vi "Configuration.vi"() -> ()   [LabVIEW 2018]
uses:
  <vilib>/Utility/miscctls.llb/LVRectTypeDef.ctl
  <vilib>/addons/database/NI_Database_API.lvlib
panel:
  in  "View":bool
  out "Headline":string
  in  "Delete Button":bool
  in  "Save Button":bool
  in  "Configuration":T1
  in  "Remark":string
  in  "Project ID":string(combo) caption="Test Name"
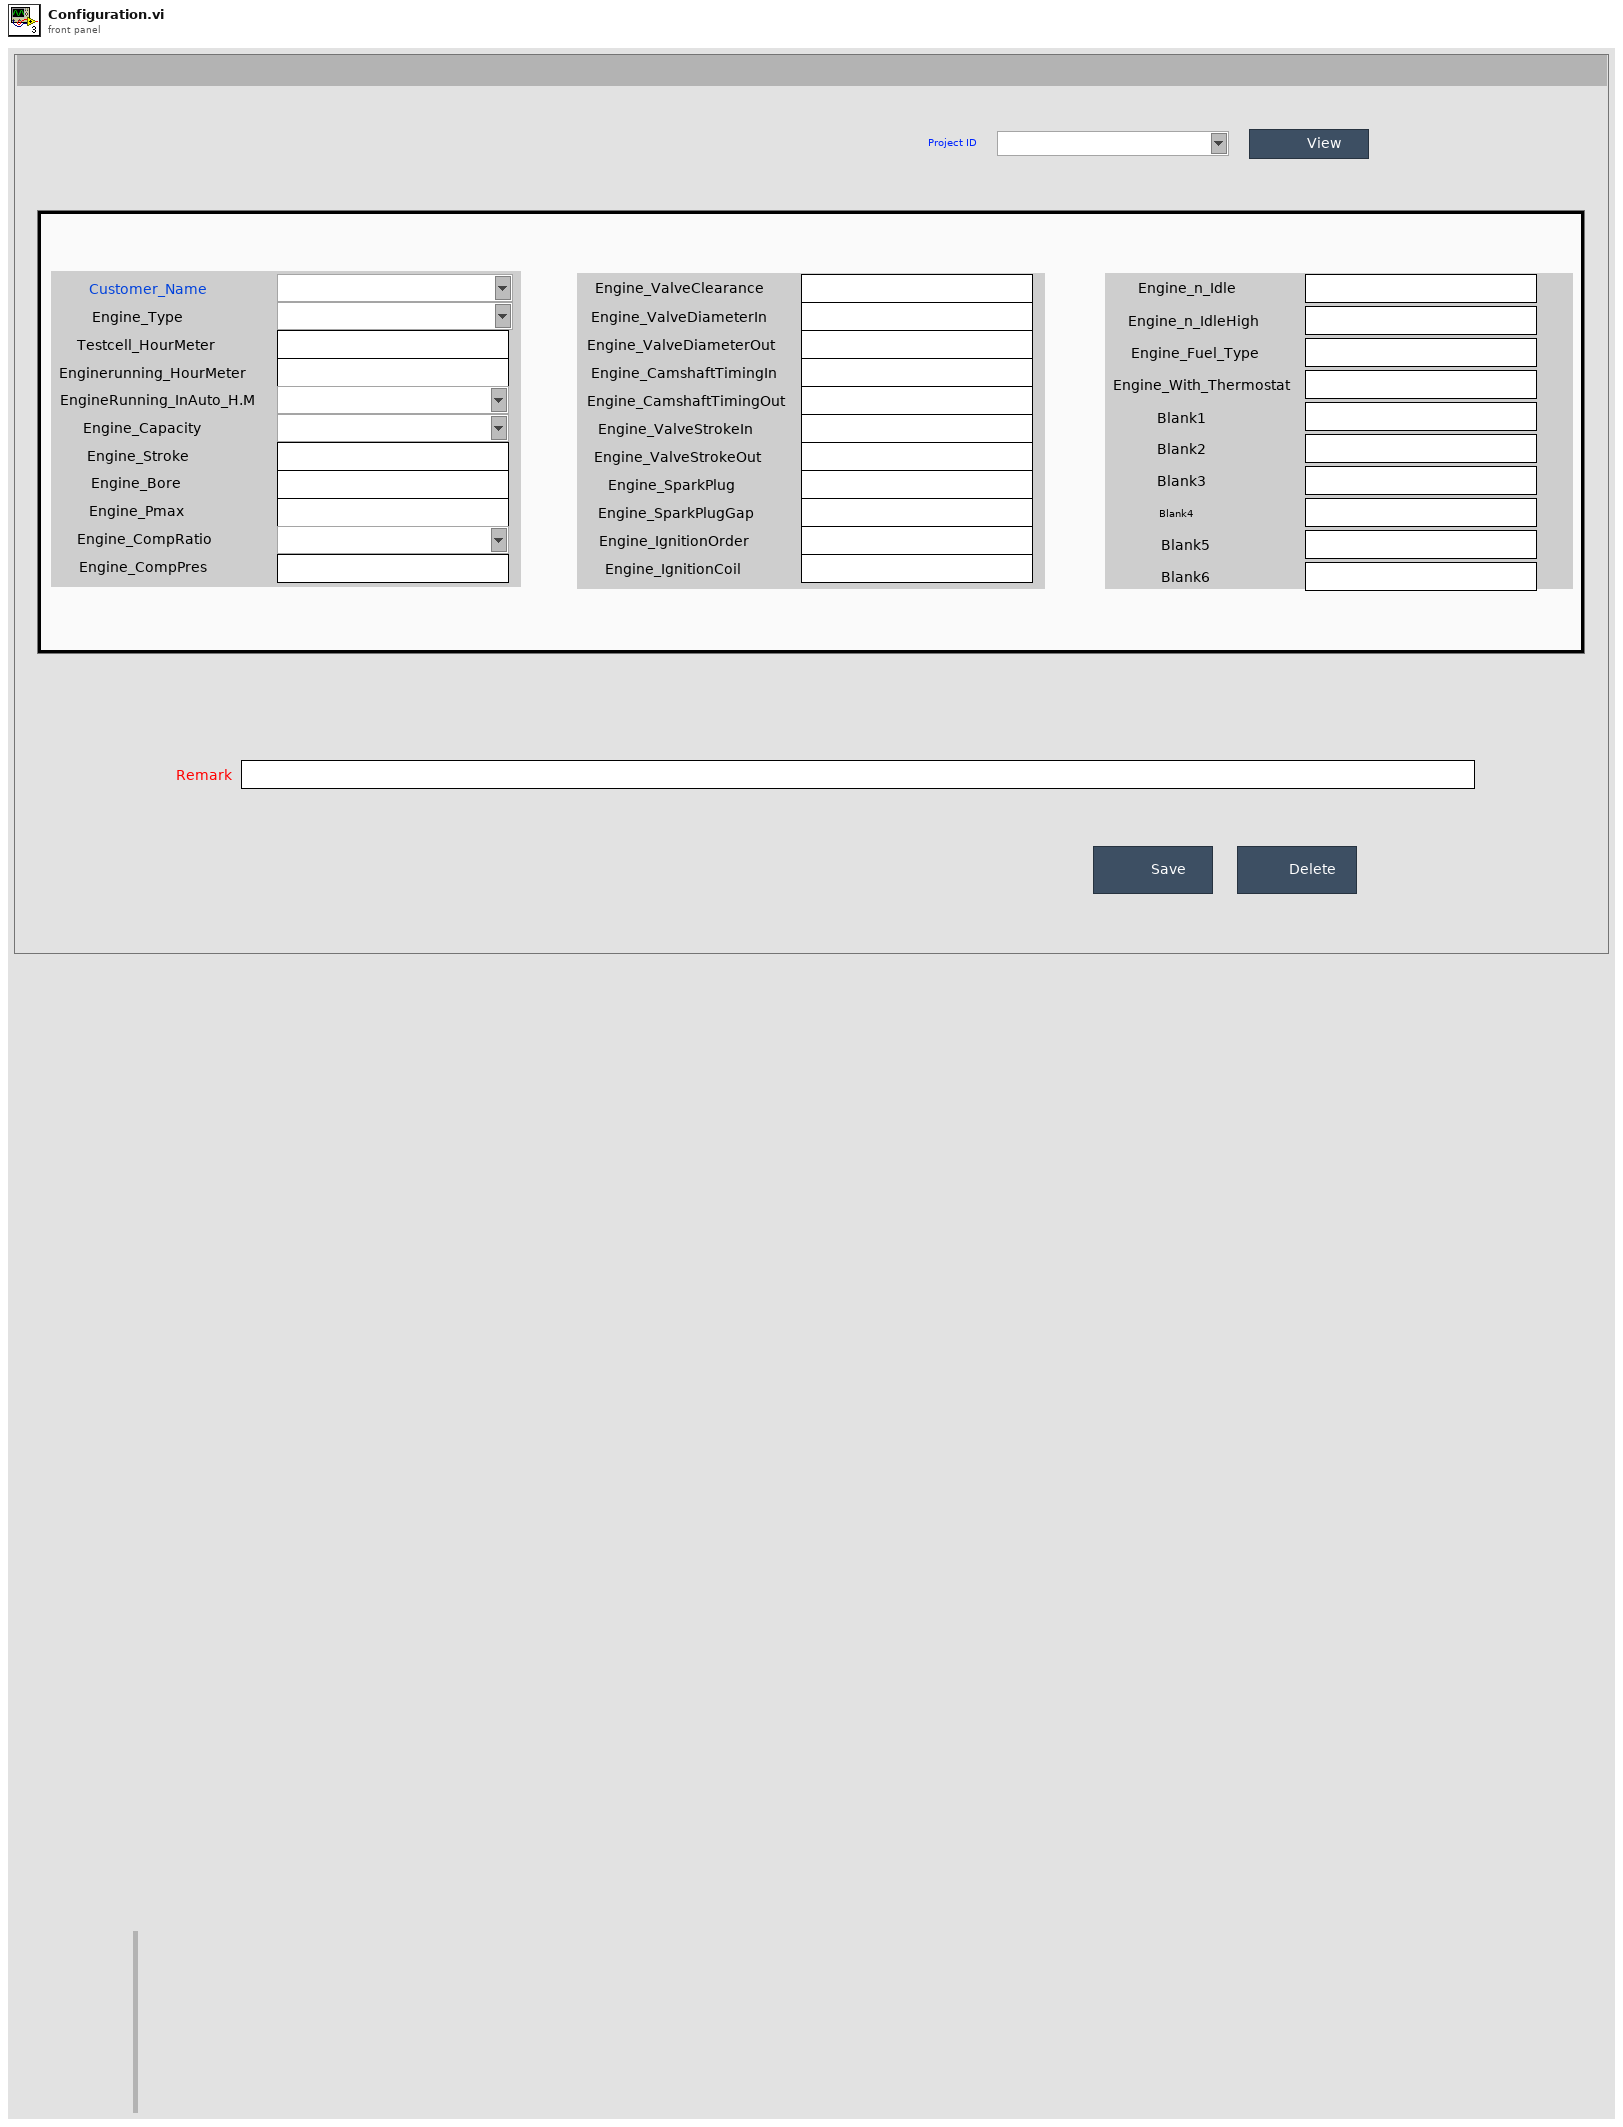
[diagram p1: front panel]
types:
  T1 = cluster{"Customer_Name":string, "Engine_Type":string, "Testcell_HourMeter":string, "Enginerunning_HourMeter":string, "EngineRunning_InAuto_H.M":string, "Engine_Capacity":string, "Engine_Stroke":string, "Engine_Bore":string, "Engine_Pmax":string, "Engine_CompRatio":string, "Engine_CompPres":string, "Engine_ValveClearance":string, "Engine_ValveDiameterIn":string, "Engine_ValveDiameterOut":string, "Engine_CamshaftTimingIn":string, "Engine_CamshaftTimingOut":string, "Engine_ValveStrokeIn":string, "Engine_ValveStrokeOut":string, "Engine_SparkPlug":string, "Engine_SparkPlugGap":string, "Engine_IgnitionOrder":string, "Engine_IgnitionCoil":string, "Engine_n_Idle":string, "Engine_n_IdleHigh":string, "Engine_Fuel_Type":string, "Engine_With_Thermostat":string, "Blank1":string, "Blank2":string, "Blank3":string, "Blank4":string, "Blank5":string, "Blank6":string}
  T2 = enum32{"Invalid", "Standard", "Closed", "Hidden", "Minimized", "Maximized"}
  T3 = enum32{"invalid app kind", "Development System", "Run Time System", "Student Edition", "Embedded LabVIEW", "Evaluation", "Custom"}
  T4 = typedef "LVRectTypeDef.ctl" = cluster{"Left":i16, "Top":i16, "Right":i16, "Bottom":i16}
  T5 = typedef "NI_Database_API.lvlib/Conn ObjectReference.ctl" = refnum<k1>
  T6 = cluster{"Core":cluster{"Current VI Reference":refnum<vi>, "Close Panel on Exit?":bool}, "Project ID":refnum<vi>, "Remark":refnum<vi>, "Controls[]":refnum<vi>[], "connection reference":T5}
  T7 = cluster{"Current VI Reference":refnum<vi>, "Close Panel on Exit?":bool}
  T8 = cluster{"[0]":string, "[1]":string, "[2]":string, "[3]":string, "[4]":string, "[5]":string, "[6]":string, "[7]":string, "[8]":string, "[9]":string, "[10]":string, "[11]":string, "[12]":string, "[13]":string, "[14]":string, "[15]":string, "[16]":string, "[17]":string, "[18]":string, "[19]":string, "[20]":string, "[21]":string, "[22]":string, "[23]":string, "[24]":string, "[25]":string, "[26]":string, "[27]":string, "[28]":string, "[29]":string, "[30]":string, "[31]":string}
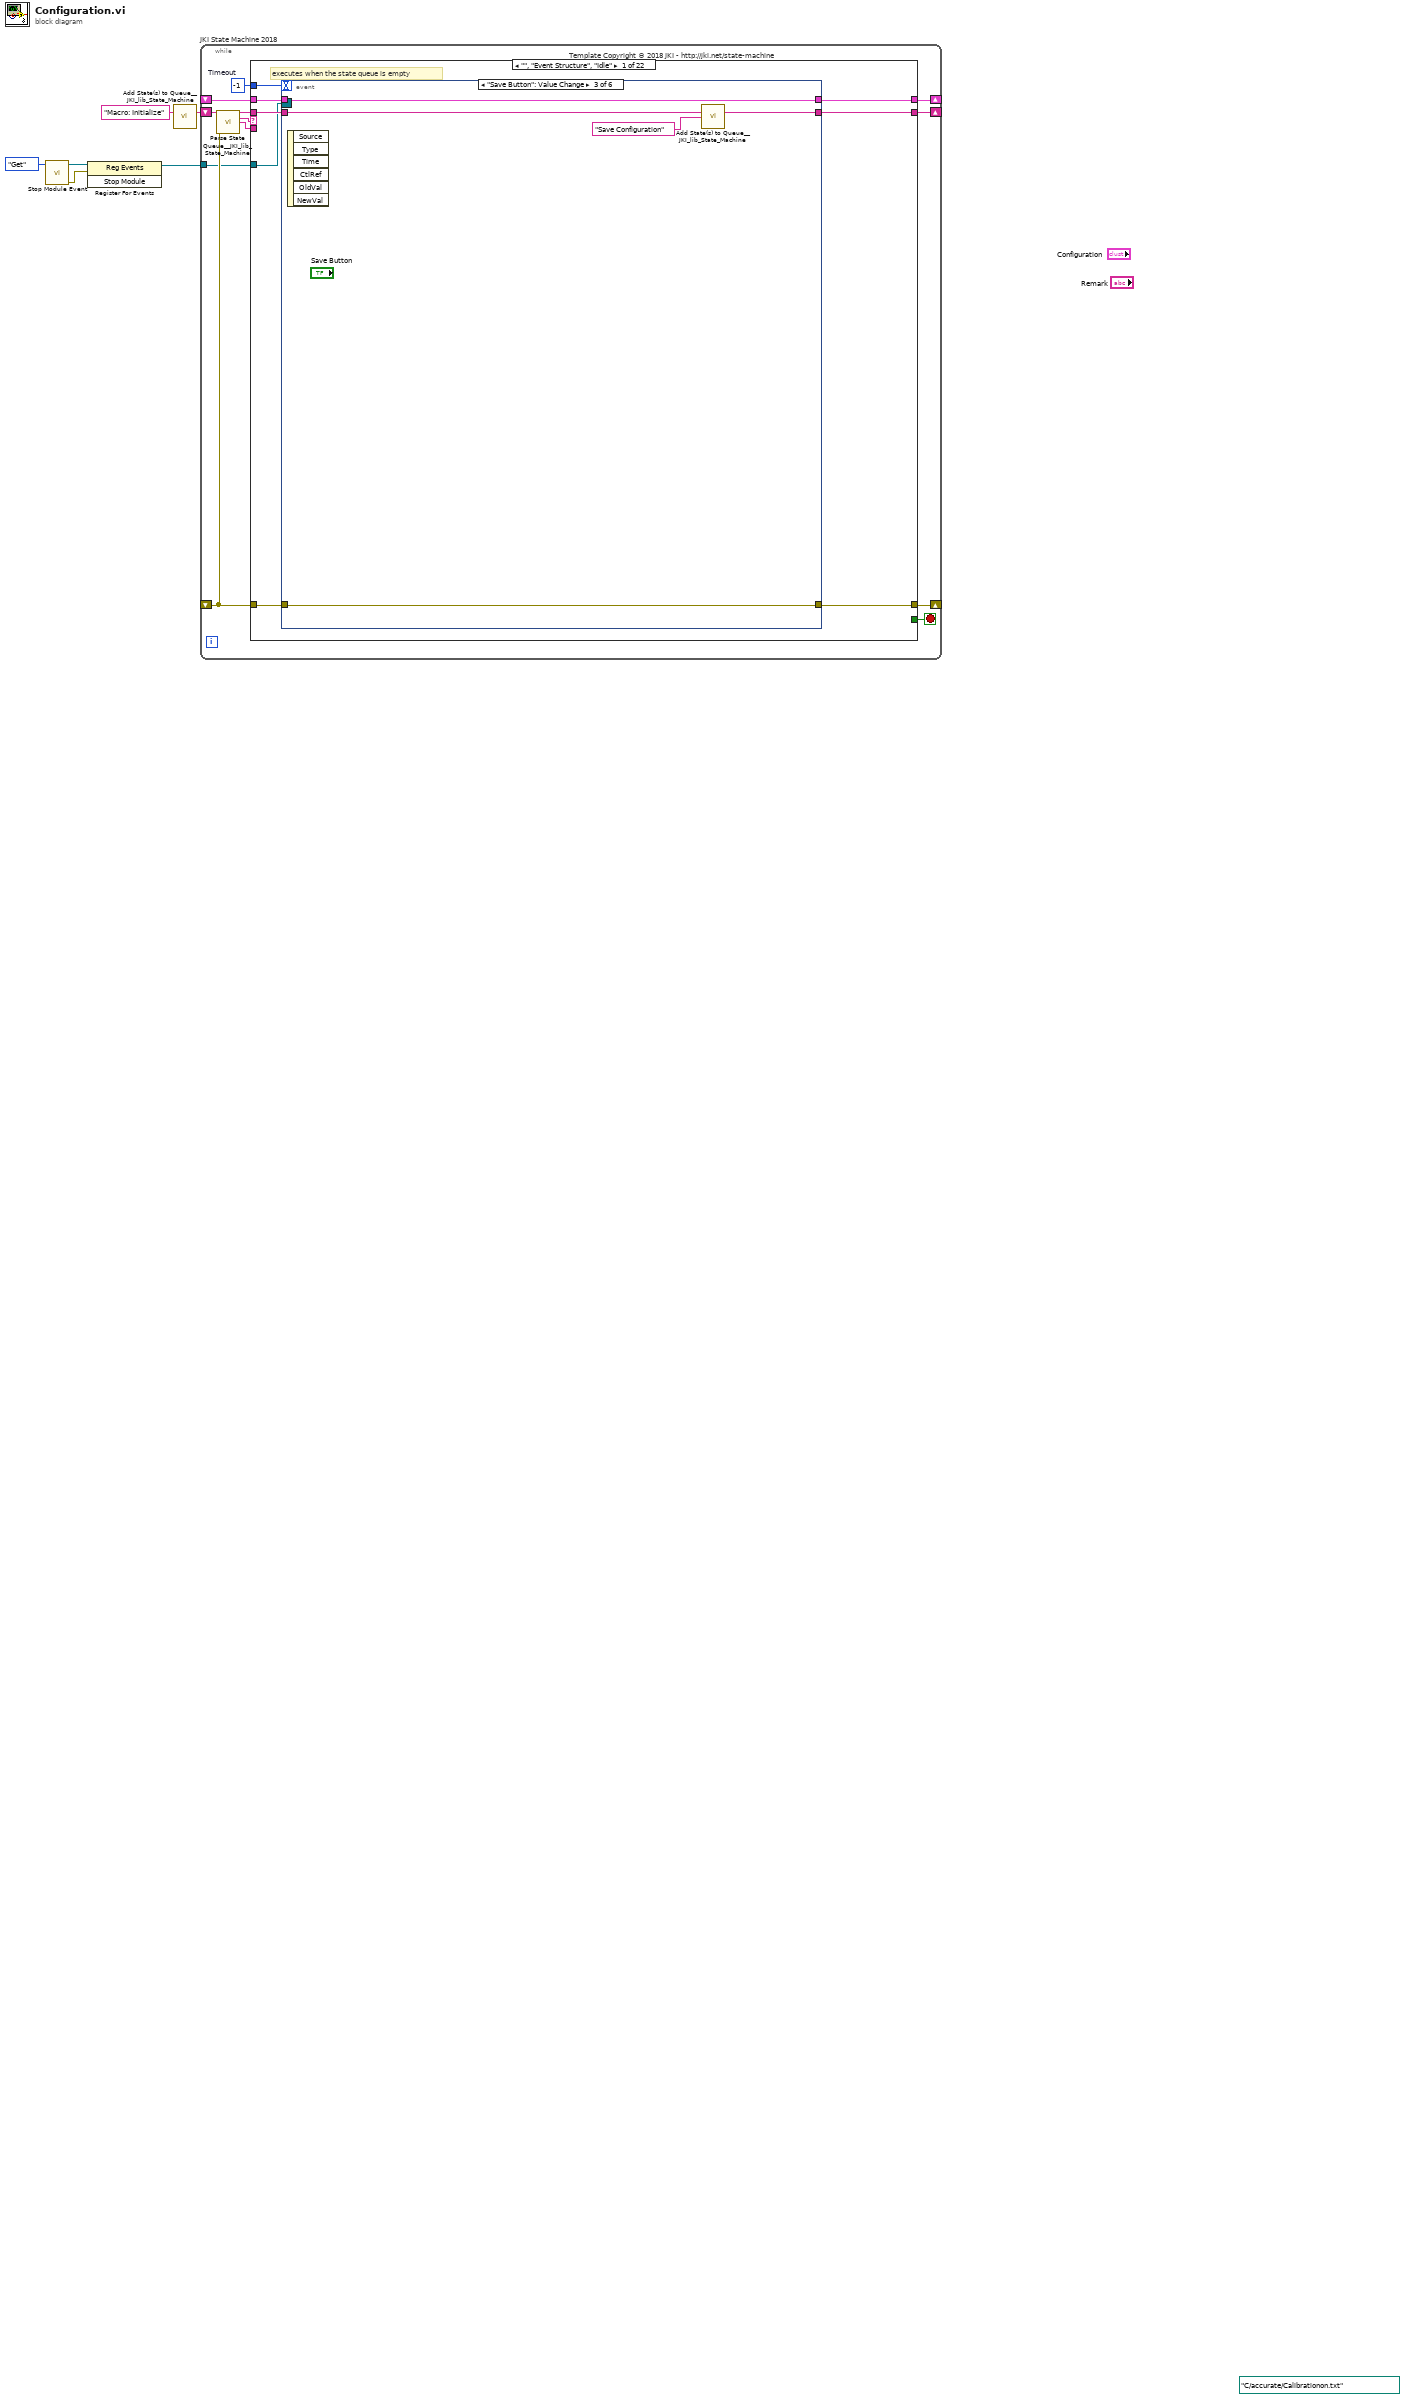
[diagram p0: block diagram]
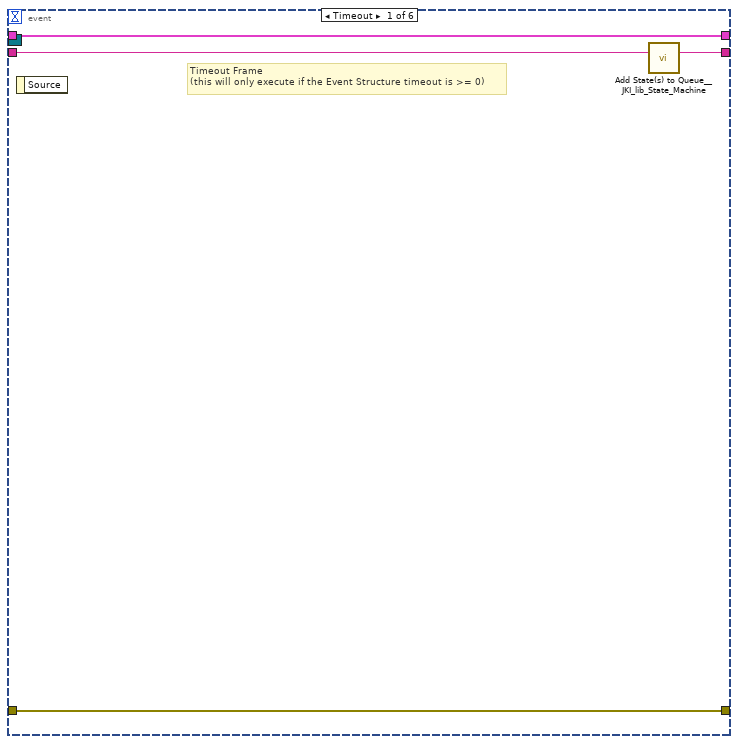
[diagram p2: hidden frame]
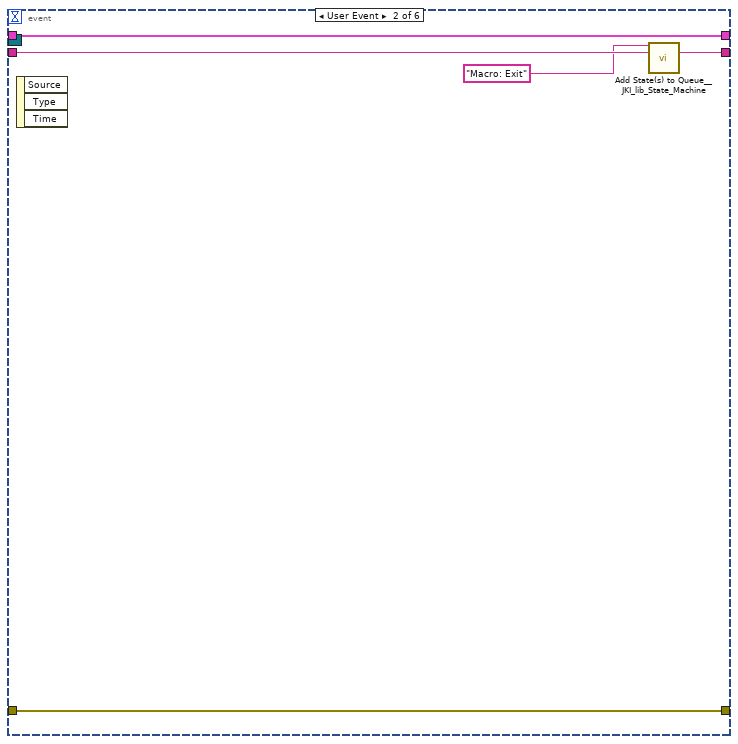
[diagram p3: hidden frame]
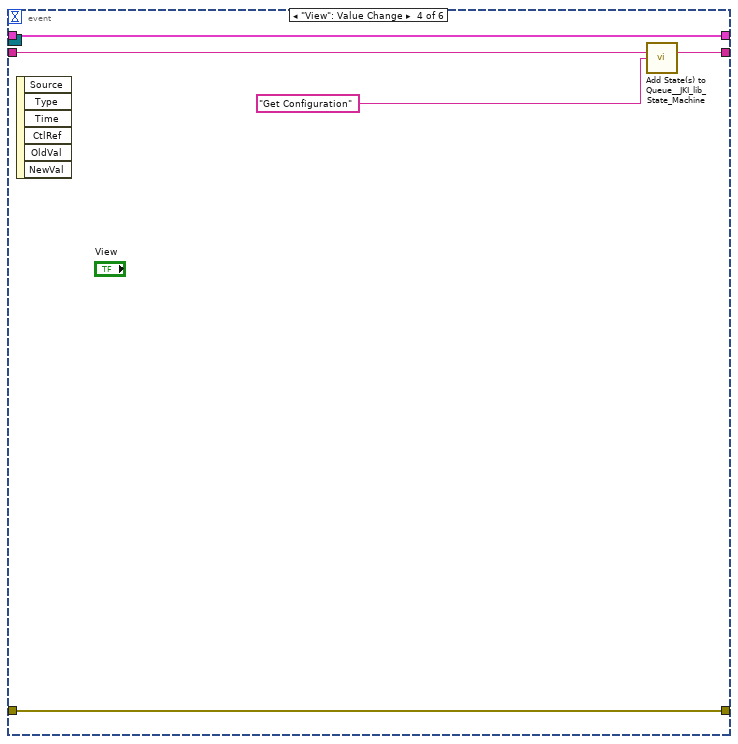
[diagram p4: hidden frame]
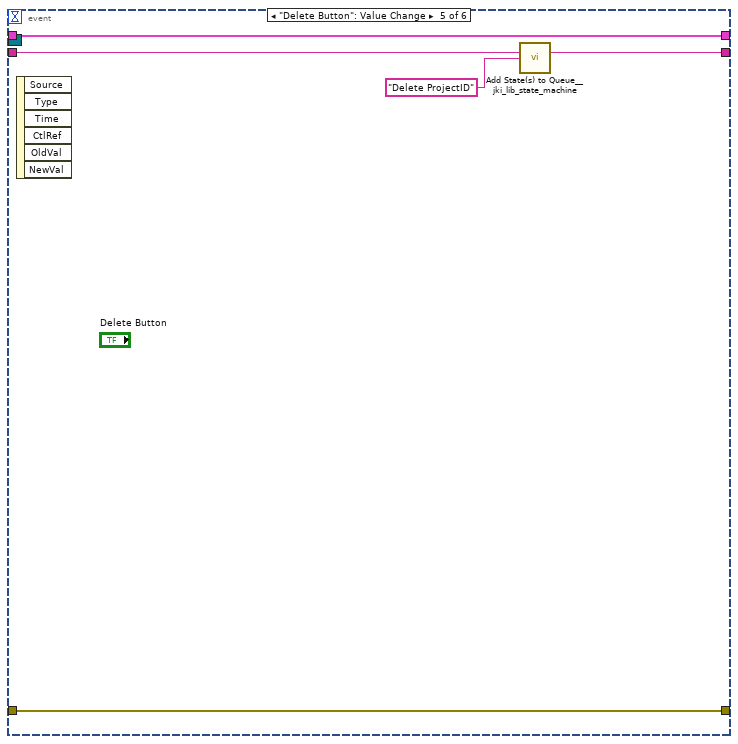
[diagram p5: hidden frame]
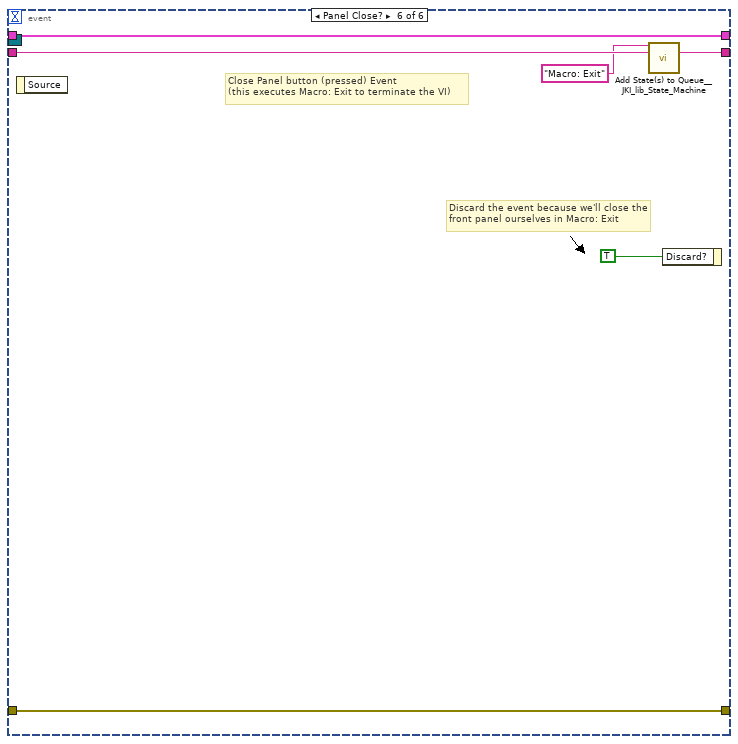
[diagram p6: hidden frame]
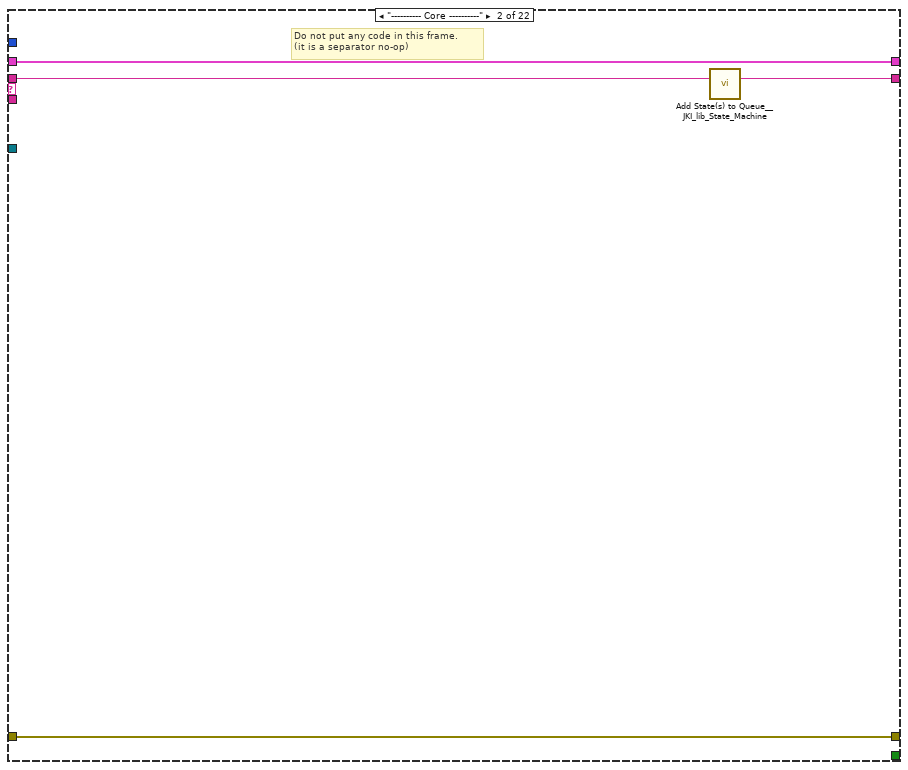
[diagram p7: hidden frame]
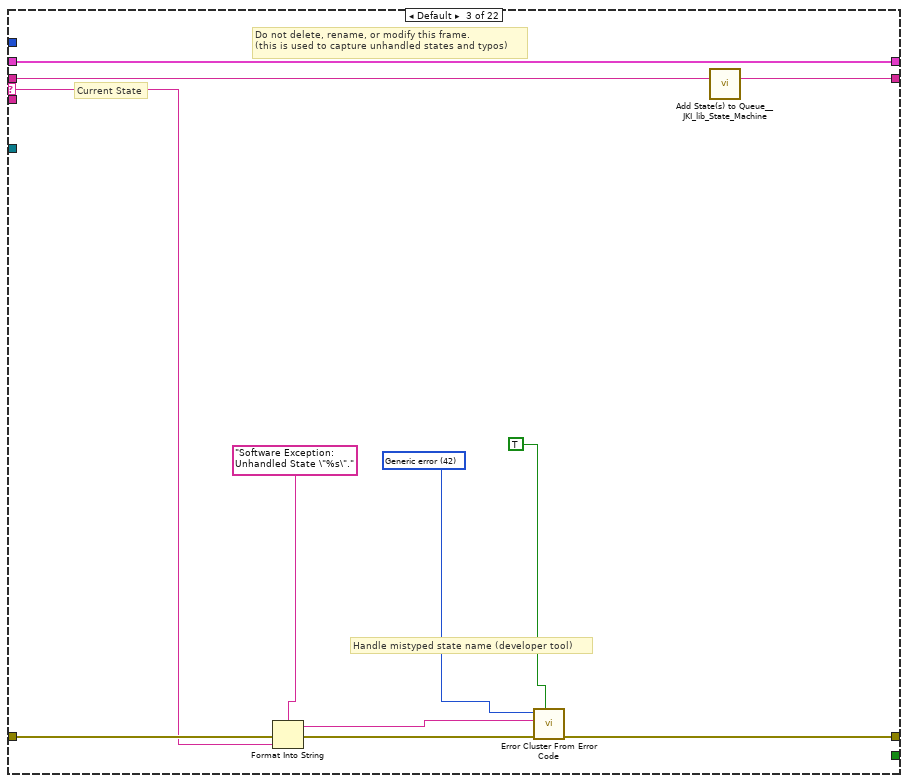
[diagram p8: hidden frame]
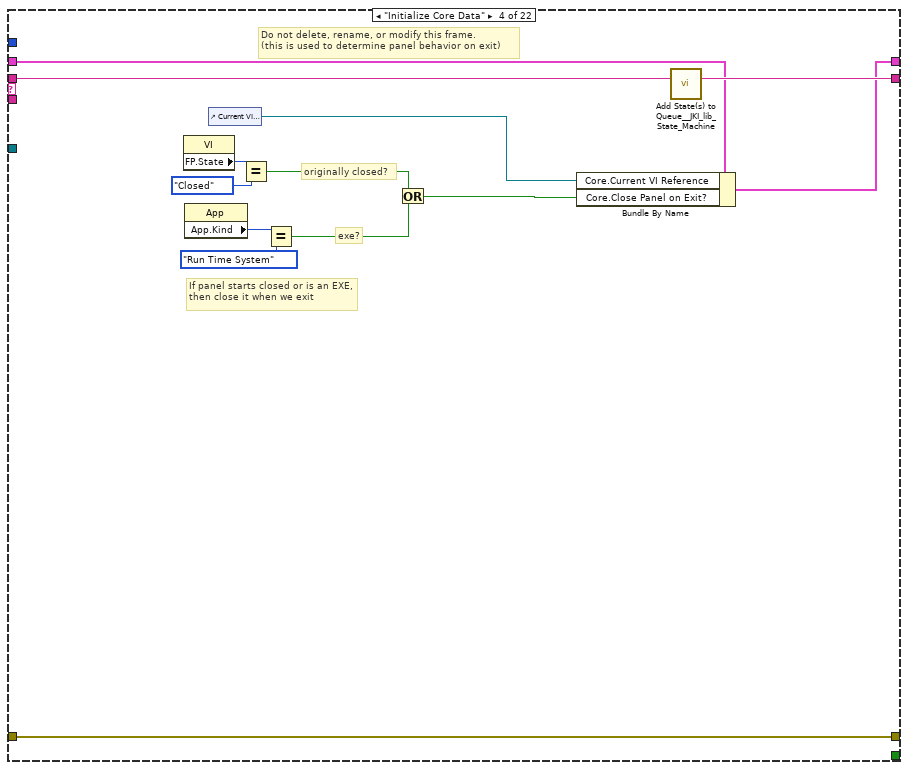
[diagram p9: hidden frame]
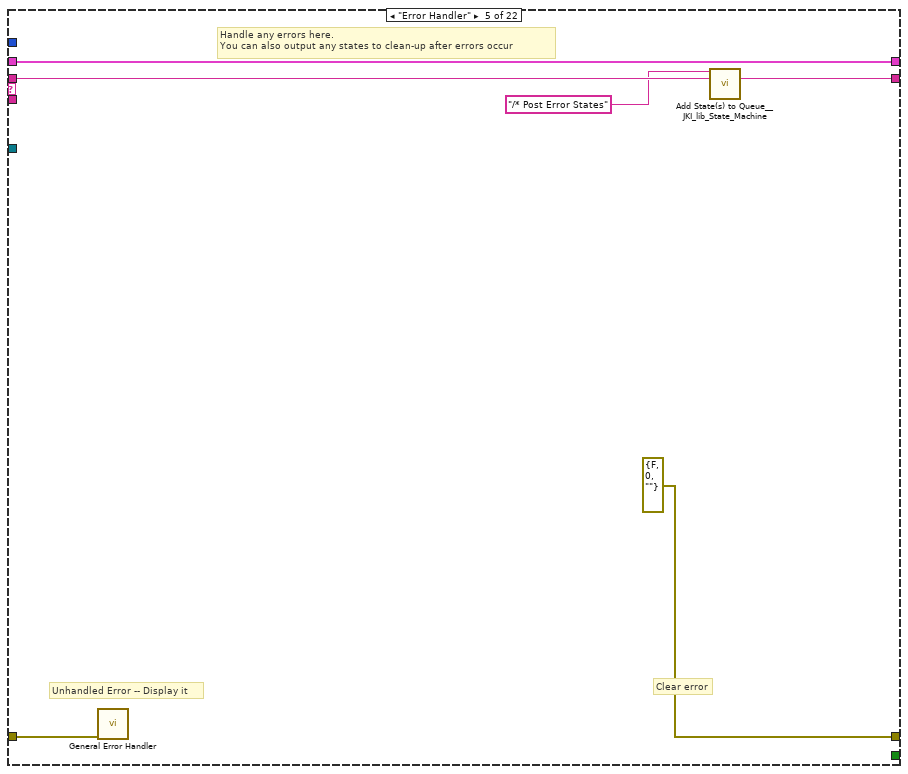
[diagram p10: hidden frame]
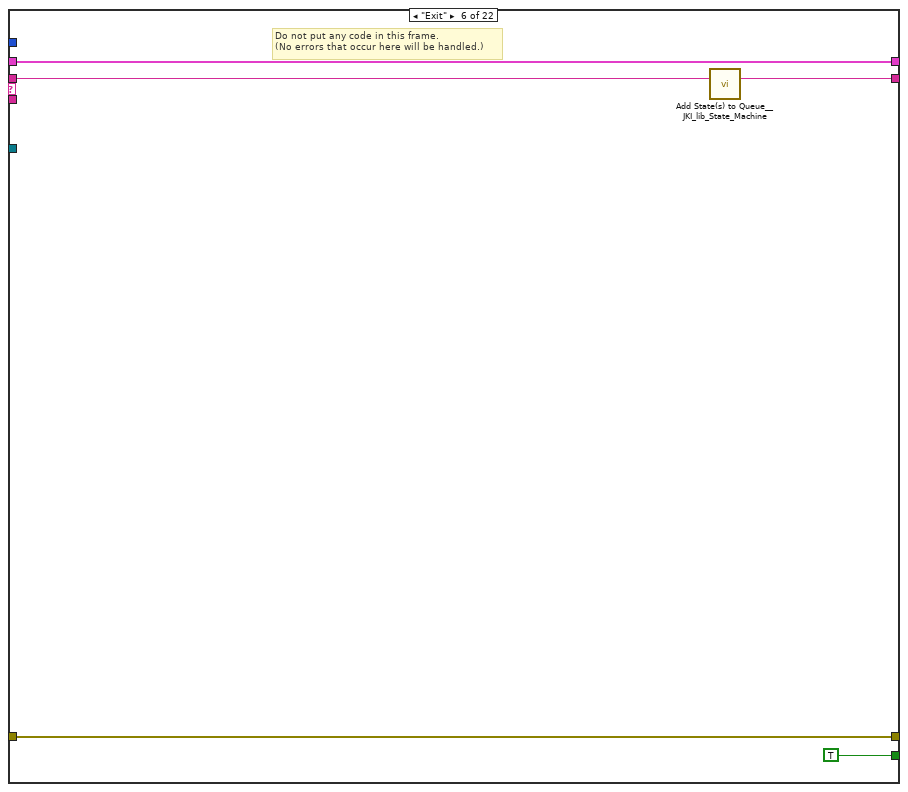
[diagram p11: hidden frame]
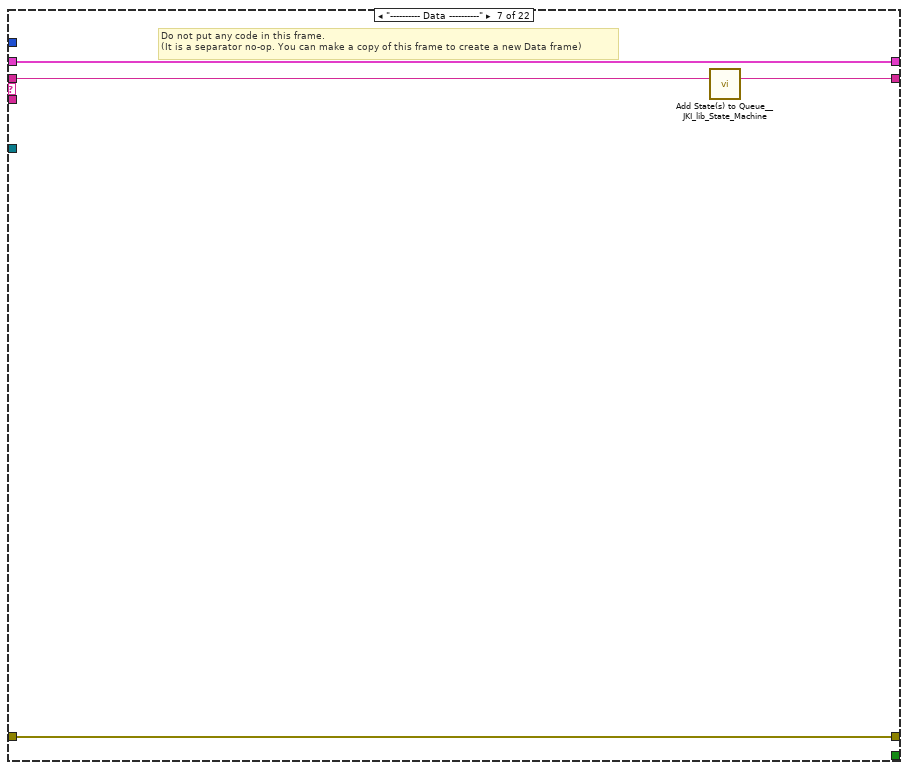
[diagram p12: hidden frame]
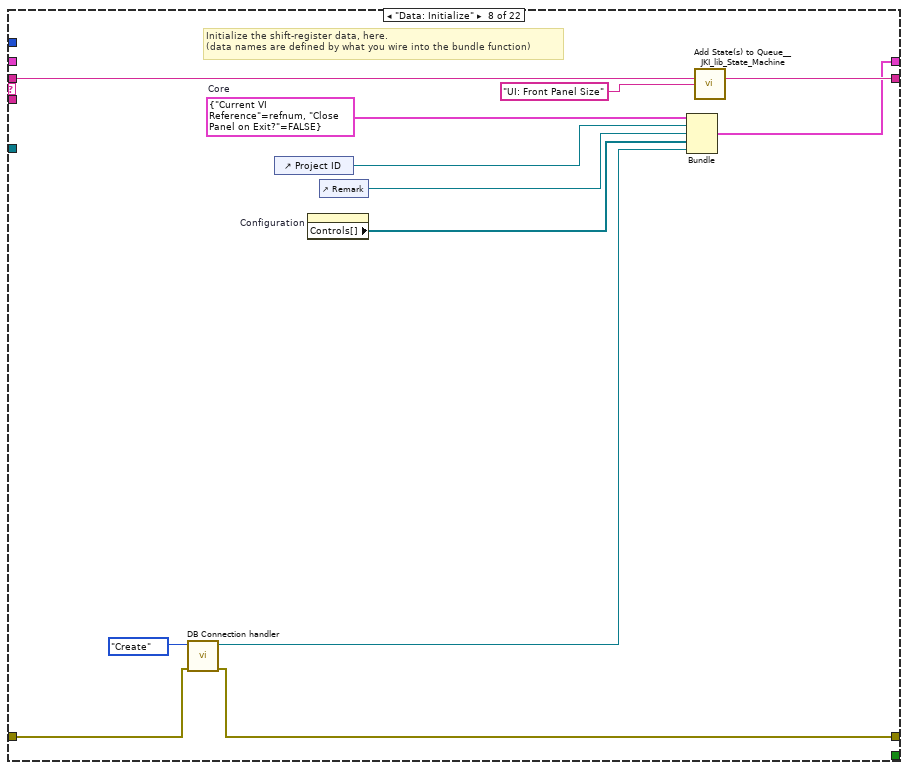
[diagram p13: hidden frame]
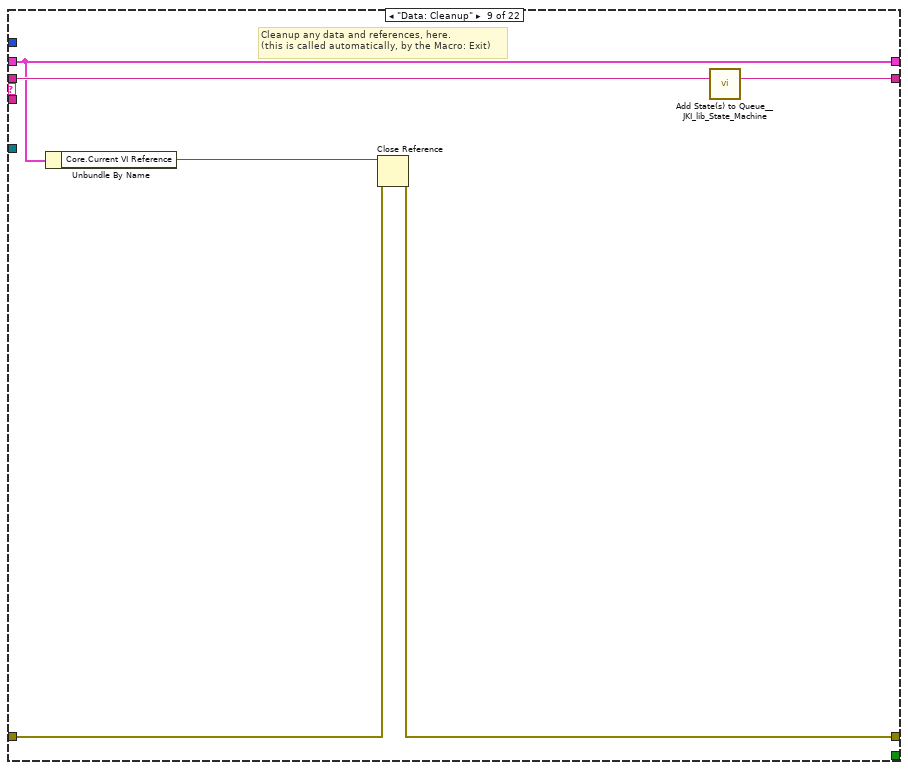
[diagram p14: hidden frame]
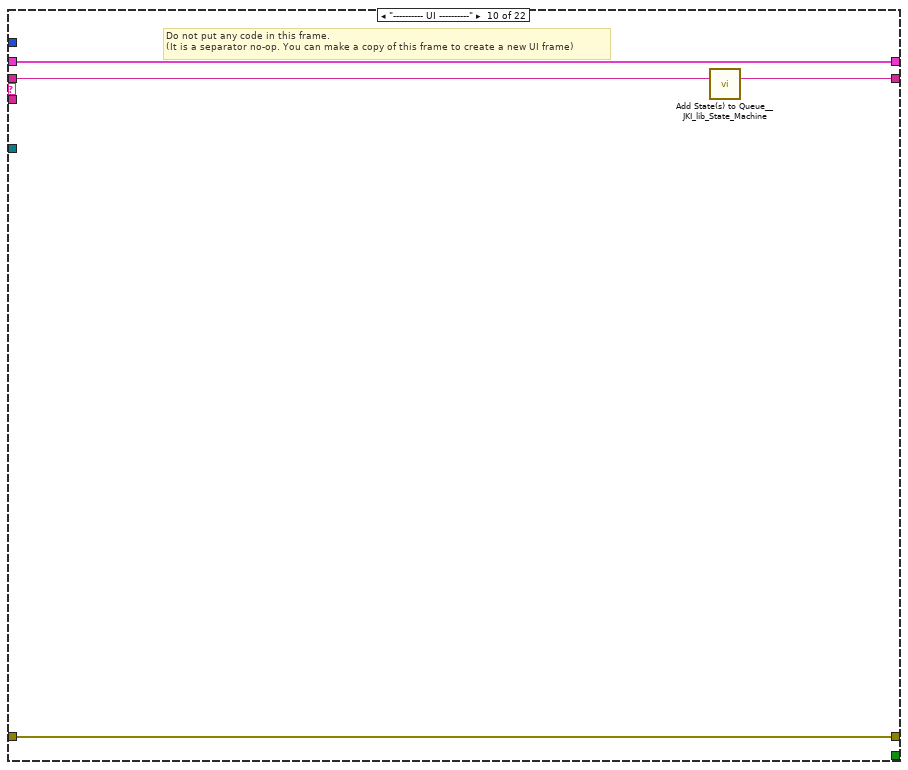
[diagram p15: hidden frame]
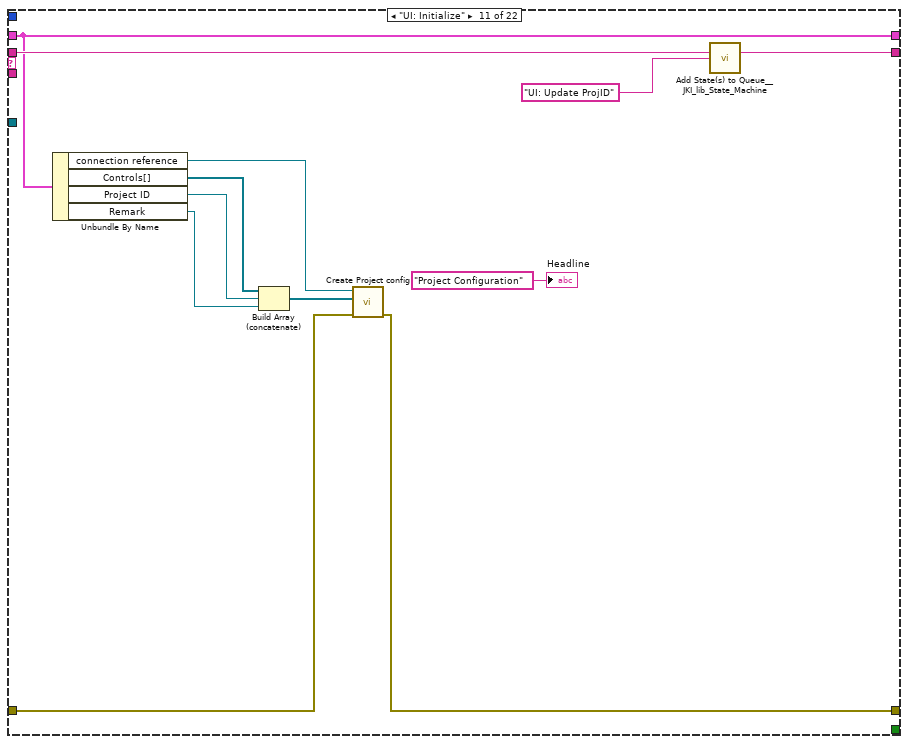
[diagram p16: hidden frame]
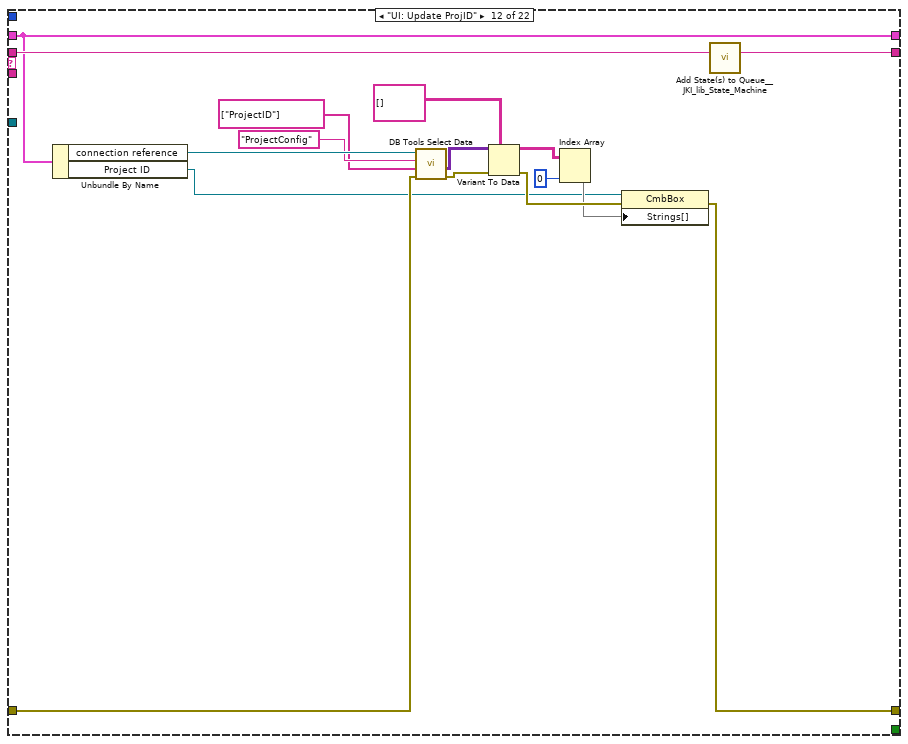
[diagram p17: hidden frame]
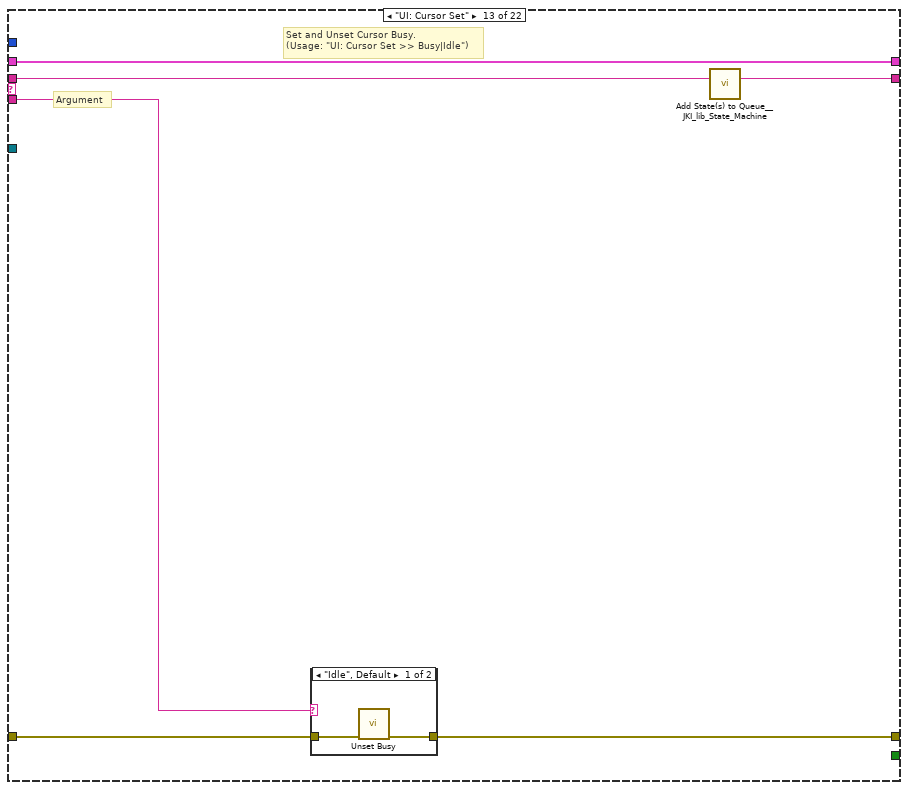
[diagram p18: hidden frame]
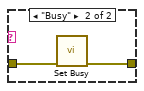
[diagram p19: hidden frame]
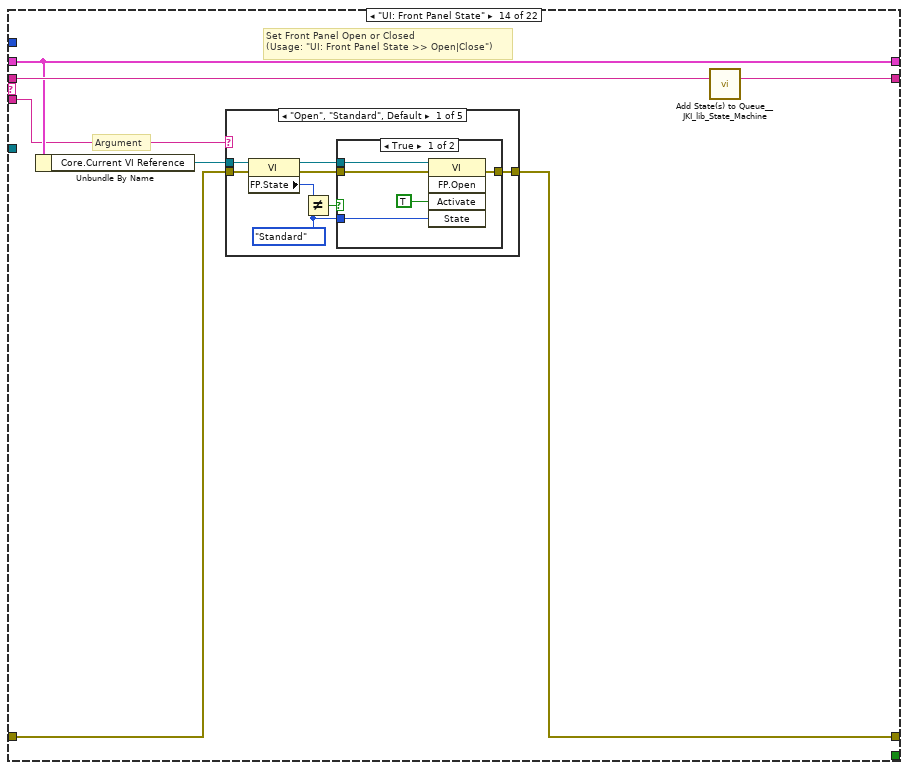
[diagram p20: hidden frame]
diagram:
  (unwired) path "C:/accurate/Calibrationon.txt" ("Dir Path In")
  n1 = call "Stop Module Event.vi"("Action"=enum16{"Create", "Get", "Destroy"}."Get") -> ("error out"=w4:errorcluster, "Stop Module"=w3:refnum<user-event>)  [unwired: 9 in]
  n2 = register-events(error in=w4, w3) -> (reference out=w2:refnum<event-registration>)  [unwired: 1 in, 1 out]
  n3 = call <vilib>:"Add State(s) to Queue__JKI_lib_State_Machine.vi"("State(s) in (\"\")"="Macro: Initialize") -> ("States Out"=w6:string)  [unwired: 14 in]
  n4 = while "JKI State Machine 2018" {
    shift-right: [w11] -> _
    shift-left: _ -> [w10]
    shift-right: [w14] -> _
    shift-left: _ -> [w8]
    shift-right: [w13] -> _
    shift-left: w6 -> [w15]
    tunnel: w2 -> [w7]
    stop <- w12 stop-if-true
    w9 = -1  # Timeout
    # "Template Copyright © 2018 JKI - http://jki.net/state-machine"
    n5 = call <vilib>:"Parse State Queue__JKI_lib_State_Machine.vi"("State Queue"=w15, "Error In (no error)"=w8) -> ("Remaining States"=w17:string, "Current State"=w18:string, "Arguments"=w16:string)  [unwired: 11 in]
    n6 = case shown="\"\", \"Event Structure\", \"Idle\"" w18 {
      selector: w18 -> [_ _ w61 _ _ _ _ _ _ _ _ _ _ _ _ _ _ _ _ _ _ _]
      tunnel: w17 -> [w26 w60 w65 w84 w90 w95 w99 w111 w117 w121 w133 w149 w155 w166 w239 w248 w253 w270 w274 w286 w316 w322]
      tunnel: w16 -> [_ _ _ _ _ _ _ _ _ _ _ _ w150 w160 _ _ _ _ _ _ _ _]
      tunnel: w10 -> [w24 w57 w63 w77 w87 w93 w96 _ w112 w118 w131 w147 w153 w162 w237 w245 w250 w268 w271 w284 w314 w324]
      tunnel: [w23 w58 w67 w81 errorcluster {"status"=FALSE, "code"=0, "source"=""} ("error out") w91 w97 w105 w113 w119 w130 w138 w151 w163 w233 w246 w251 w255 w272 w275 w304 w320] -> w14
      tunnel: w8 -> [w22 w58 w66 w81 w86 w91 w97 w106 w114 w119 w129 w135 w152 w164 w234 w246 w251 w260 w272 w283 w308 w318]
      tunnel: [w25 w59 w64 w83 w89 w94 w98 w110 w116 w120 w132 w148 w154 w165 w238 w247 w252 w269 w273 w285 w315 w323] -> w13
      tunnel: [_ _ _ _ _ TRUE _ _ _ _ _ _ _ _ _ _ _ _ _ _ _ _] -> w12
      tunnel: [w21 w57 w63 w82 w87 w93 w96 w109 w112 w118 w131 w147 w153 w162 w237 w245 w250 w268 w271 w284 w314 w324] -> w11
      tunnel: w9 -> [w20 _ _ _ _ _ _ _ _ _ _ _ _ _ _ _ _ _ _ _ _ _]
      tunnel: w7 -> [w19 _ _ _ _ _ _ _ _ _ _ _ _ _ _ _ _ w261 _ _ _ _]
      frame "", "Event Structure", "Idle" {
        # "executes when the state queue is empty"
        n7 = event shown="[2] \"Save Button\": Value Change" {
          selector: w19 -> [_ _ _ _ _ _]
          dyn-events: _ -> [_ _ _ _ _ _]
          timeout: w20 -> [_ _ _ _ _ _]
          tunnel: w26 -> [w30 w35 w38 w43 w47 w56]
          tunnel: [w29 w34 w39 w44 w48 w55] -> w25
          tunnel: w24 -> [w27 w32 w40 w45 w49 w53]
          tunnel: [w28 w33 w36 w41 w50 w54] -> w23
          tunnel: w22 -> [w28 w33 w36 w41 w50 w54]
          tunnel: [w27 w32 w40 w45 w49 w53] -> w21
          event Timeout {
            # "Timeout Frame\n(this will only execute if the Event Structure timeout is >= 0)"
            n8 = event-data() -> ()  [unwired: 1 in, 1 out]
            n9 = call <vilib>:"Add State(s) to Queue__JKI_lib_State_Machine.vi"("State(s) in (\"\")"=w30) -> ("States Out"=w29:string)  [unwired: 14 in]
          }
          event User Event {
            n10 = event-data() -> ()  [unwired: 1 in, 3 out]
            n11 = call <vilib>:"Add State(s) to Queue__JKI_lib_State_Machine.vi"("State(s) in Front (\"\")"="Macro: Exit", "State(s) in (\"\")"=w35) -> ("States Out"=w34:string)  [unwired: 13 in]
          }
          event "Save Button": Value Change {
            n12 = event-data() -> ()  [unwired: 1 in, 6 out]
            n13 = call <vilib>:"Add State(s) to Queue__JKI_lib_State_Machine.vi"("State(s) in (\"\")"=w38, "State(s) at Back (\"\")"="Save Configuration" ("State(s) at Back (\"\")")) -> ("States Out"=w39:string)  [unwired: 13 in]
          }
          event "View": Value Change {
            n14 = event-data() -> ()  [unwired: 1 in, 6 out]
            n15 = call <vilib>:"Add State(s) to Queue__JKI_lib_State_Machine.vi"("State(s) in (\"\")"=w43, "State(s) at Back (\"\")"="Get Configuration" ("State(s) at Back (\"\")")) -> ("States Out"=w44:string)  [unwired: 13 in]
          }
          event "Delete Button": Value Change {
            n16 = event-data() -> ()  [unwired: 1 in, 6 out]
            n17 = call <vilib>:"Add State(s) to Queue__jki_lib_state_machine.vi"("State(s) in (\"\")"=w47, "State(s) at Back (\"\")"="Delete ProjectID" ("State(s) at Back (\"\")")) -> ("States Out"=w48:string)  [unwired: 13 in]
          }
          event Panel Close? {
            # "Discard the event because we'll close the front panel ourselves in Macro: Exit"
            # "Close Panel button (pressed) Event\n(this executes Macro: Exit to terminate the VI)"
            n18 = event-data() -> ()  [unwired: 1 in, 1 out]
            n19 = call <vilib>:"Add State(s) to Queue__JKI_lib_State_Machine.vi"("State(s) in Front (\"\")"="Macro: Exit", "State(s) in (\"\")"=w56) -> ("States Out"=w55:string)  [unwired: 13 in]
            n20 = event-data("Discard?"=TRUE) -> ()  [unwired: 1 in, 1 out]
          }
        }
      }
      frame "---------- Core ----------" {
        # "Do not put any code in this frame.\n(it is a separator no-op)"
        n21 = call <vilib>:"Add State(s) to Queue__JKI_lib_State_Machine.vi"("State(s) in (\"\")"=w60) -> ("States Out"=w59:string)  [unwired: 14 in]
      }
      frame Default {
        w70 = 42 items=["No error", "Argument error", "Memory is full", "Out of zone", "End of file", "File already open", "Generic file I/O error", "File not found", "File permission error", "Disk is full", "Duplicate path", "Too many files open", "System feature not enabled", "Resource file not found", "Cannot add resource", "Resource not found", "Image not found", "Image memory error", "Pen does not exist", "Config type invalid", "Config token not found", "Config parse error", "Config memory error", "Bad external code format", "Bad external code offset", "External code not present", "Null window", "Destroy window error", "Null menu", "Print aborted", "Bad print record", "Print driver error", "Windows error during printing", "Memory error during printing", "Print dialog error", "Generic print error", "Invalid device refnum", "Device not found", "Device parameter error", "Device unit error", "Cannot open device", "Device call aborted", "Generic error", "Cancelled by user", "Object ID too low", "Object ID too high", "Object not in heap", "Unknown heap", "Unknown object (invalid DefProc)", "Unknown object (DefProc not in table)", "Message out of range", "Invalid (null) method", "Unknown message", "Manager call not supported", "Bad address", "Network operation in progress", "Network operation timed out", "Connection is busy", "Network attribute not supported", "Network error", "Address in use", "System out of memory", "Connection aborted", "Connection refused", "Not connected", "Already connected", "Connection closed", "Initialization error (interapplication manager)", "Bad occurrence", "Wait on unbound occurrence handler", "Occurrence queue overflow", "Datalog type conflict", "Unused", "Unrecognized type (interapplication manager)", "Memory corrupt", "Failed to make temporary DLL", "Old CIN version", "Drag socket not found", "Failed to load drop-object", "Failed to register OLE object", "Failed to release OLE object", "Format specifier type mismatch", "Unknown format specifier", "Too few format specifiers", "Too many format specifiers", "Scan failed", "Newer CIN version", "Error converting to variant", "Runtime menu error", "Password tampered", "Variant attribute not found", "Incompatible variant data type", "Event data is not available", "Event Store is not present", "Occurrence is not found", "Event Queue is not created", "Event info is not available", "Refnum passed is NULL", "Error retrieving Class GUID", "Error retrieving CoClass GUID", "Error retrieving TypeLib GUID.", "Bad built application magic bytes.", "Specific driver is different from the specific driver associated with the Logical Name.", "There is no session opened to the class driver.", "Max Error", "MAX - Error with config objects", "MAX - Error loading configuration", "MAX - Group not supported"]
        # "Current State"
        # "Do not delete, rename, or modify this frame.\n(this is used to capture unhandled states and typos)"
        # "Handle mistyped state name (developer tool)"
        n22 = Format Into String(format string="Software Exception: Unhandled State \"%s\"." ("message"), error in=w66, w61) -> (resulting string=w69:string, error out=w68:errorcluster)  [unwired: 1 in]
        n23 = call <vilib>:"Error Cluster From Error Code.vi"("show call chain? (False)"=TRUE, "error in (no error)"=w68, "error message (\"\")"=w69, "error code (0)"=w70) -> ("error out"=w67:errorcluster)  [unwired: 5 in]
        n24 = call <vilib>:"Add State(s) to Queue__JKI_lib_State_Machine.vi"("State(s) in (\"\")"=w65) -> ("States Out"=w64:string)  [unwired: 14 in]
      }
      frame "Initialize Core Data" {
        # "Do not delete, rename, or modify this frame.\n(this is used to determine panel behavior on exit)"
        # "originally closed?"
        # "exe?"
        # "If panel starts closed or is an EXE, then close it when we exit"
        n25 = property class="VI"() -> ("FP.State"=w74:T2)  [unwired: 2 in, 2 out]
        n26 = property class="App"() -> ("App.Kind"=w80:T3)  [unwired: 2 in, 2 out]
        n27 = control-ref of="Current VI Reference"() -> (w75:refnum<vi>)
        n28 = Equal?(x=w74, y=T2."Closed" ("Front Panel Window:State")) -> (x = y?=w72:bool)
        n29 = Equal?(x=w80, y=T3."Run Time System" ("Application:Kind")) -> (x = y?=w78:bool)
        n30 = Or(x=w72, y=w78) -> (x .or. y?=w76:bool)
        n31 = Bundle By Name(cluster=w77, "Core.Current VI Reference"=w75, "Core.Close Panel on Exit?"=w76) -> (w82:T6)
        n32 = call <vilib>:"Add State(s) to Queue__JKI_lib_State_Machine.vi"("State(s) in (\"\")"=w84) -> ("States Out"=w83:string)  [unwired: 14 in]
      }
      frame "Error Handler" {
        # "Unhandled Error -- Display it"
        # "Handle any errors here.\nYou can also output any states to clean-up after errors occur"
        # "Clear error"
        n33 = call <vilib>:"General Error Handler.vi"("error in (no error)"=w86) -> ()  [unwired: 10 in, 5 out]
        n34 = call <vilib>:"Add State(s) to Queue__JKI_lib_State_Machine.vi"("State(s) in Front (\"\")"="/* Post Error States", "State(s) in (\"\")"=w90) -> ("States Out"=w89:string)  [unwired: 13 in]
      }
      frame "Exit" {
        # "Do not put any code in this frame.\n(No errors that occur here will be handled.)"
        n35 = call <vilib>:"Add State(s) to Queue__JKI_lib_State_Machine.vi"("State(s) in (\"\")"=w95) -> ("States Out"=w94:string)  [unwired: 14 in]
      }
      frame "---------- Data ----------" {
        # "Do not put any code in this frame.\n(It is a separator no-op. You can make a copy of this frame to create a new Data frame)"
        n36 = call <vilib>:"Add State(s) to Queue__JKI_lib_State_Machine.vi"("State(s) in (\"\")"=w99) -> ("States Out"=w98:string)  [unwired: 14 in]
      }
      frame "Data: Initialize" {
        w108 = T7 {"Current VI Reference"=refnum, "Close Panel on Exit?"=FALSE}  # Core
        # "Initialize the shift-register data, here.\n(data names are defined by what you wire into the bundle function)"
        n37 = call "DB Connection handler.vi"("error in (no error)"=w106, "DB Action"=enum16{"Create", "Close", "Get"}."Create") -> ("error out"=w105:errorcluster, "connection reference"=w104:T5)  [unwired: 8 in]
        n38 = control-ref of="Project ID"() -> (w103:refnum<vi>)
        n39 = property on="Configuration" class="Clust (strict)"() -> ("Controls[]"=w101:refnum<vi>[])  [unwired: 2 in, 2 out]
        n40 = control-ref of="Remark"() -> (w102:refnum<vi>)
        n41 = Bundle("Core"=w108, "Project ID"=w103, "Remark"=w102, "Controls[]"=w101, "connection reference"=w104) -> (w109:T6)  [unwired: 1 in]
        n42 = call <vilib>:"Add State(s) to Queue__JKI_lib_State_Machine.vi"("State(s) in (\"\")"=w111, "State(s) at Back (\"\")"="UI: Front Panel Size" ("State(s) at Back (\"\")")) -> ("States Out"=w110:string)  [unwired: 13 in]
      }
      frame "Data: Cleanup" {
        # "Cleanup any data and references, here.\n(this is called automatically, by the Macro: Exit)"
        n43 = Unbundle By Name(w112) -> ("Core.Current VI Reference"=w115:refnum<vi>)
        n44 = Close Reference(reference=w115, error in (no error)=w114) -> (error out=w113:errorcluster)
        n45 = call <vilib>:"Add State(s) to Queue__JKI_lib_State_Machine.vi"("State(s) in (\"\")"=w117) -> ("States Out"=w116:string)  [unwired: 14 in]
      }
      frame "---------- UI ----------" {
        # "Do not put any code in this frame.\n(It is a separator no-op. You can make a copy of this frame to create a new UI frame)"
        n46 = call <vilib>:"Add State(s) to Queue__JKI_lib_State_Machine.vi"("State(s) in (\"\")"=w121) -> ("States Out"=w120:string)  [unwired: 14 in]
      }
      frame "UI: Initialize" {
        n47 = Unbundle By Name(w131) -> ("connection reference"=w128:T5, "Controls[]"=w126:refnum<vi>[], "Project ID"=w125:refnum<vi>, "Remark"=w124:refnum<vi>)
        n48 = Build Array (concatenate)(w126, w125, w124) -> (w127:refnum<vi>[])
        n49 = call "Create Project config.vi"("error in (no error)"=w129, "Array"=w127, "Refnum in"=w128) -> ("error out"=w130:errorcluster)  [unwired: 8 in]
        n50 = call <vilib>:"Add State(s) to Queue__JKI_lib_State_Machine.vi"("State(s) in (\"\")"=w133, "State(s) at Back (\"\")"="UI: Update ProjID" ("State(s) at Back (\"\")")) -> ("States Out"=w132:string)  [unwired: 13 in]
        "Headline" <- "Project Configuration" ("Headline")
      }
      frame "UI: Update ProjID" {
        n51 = Unbundle By Name(w147) -> ("connection reference"=w146:T5, "Project ID"=w134:refnum<vi>)
        n52 = call <vilib>:"DB Tools Select Data.vi"("error in (no error)"=w135, "columns"=string[] ["ProjectID"], "table"="ProjectConfig", "connection reference"=w146) -> ("error out"=w142:errorcluster, "data"=w144:variant[][])  [unwired: 2 in, 1 out]
        n53 = Variant To Data(error in=w142, type=string[][] [], Variant=w144) -> (data=w141:string[][], error out=w140:errorcluster)
        n54 = Index Array(array=w141, index (col)=0 ("index (row)")) -> (element=w139:string[])  [unwired: 1 in]
        n55 = property class="CmbBox"(reference=w134, error in=w140, "Strings[]"=w139) -> (error out=w138:errorcluster)  [unwired: 1 out]
        n56 = call <vilib>:"Add State(s) to Queue__JKI_lib_State_Machine.vi"("State(s) in (\"\")"=w149) -> ("States Out"=w148:string)  [unwired: 14 in]
      }
      frame "UI: Cursor Set" {
        # "Argument"
        # "Set and Unset Cursor Busy.\n(Usage: \"UI: Cursor Set >> Busy|Idle\")"
        n57 = case shown="\"Idle\", Default" w150 {
          tunnel: w152 -> [w157 w159]
          tunnel: [w156 w158] -> w151
          frame "Idle", Default {
            n58 = call <vilib>:"Unset Busy.vi"("error in (no error)"=w157) -> ("error out"=w156:errorcluster)  [unwired: 10 in]
          }
          frame "Busy" {
            n59 = call <vilib>:"Set Busy.vi"("error in (no error)"=w159) -> ("error out"=w158:errorcluster)  [unwired: 9 in, 1 out]
          }
        }
        n60 = call <vilib>:"Add State(s) to Queue__JKI_lib_State_Machine.vi"("State(s) in (\"\")"=w155) -> ("States Out"=w154:string)  [unwired: 14 in]
      }
      frame "UI: Front Panel State" {
        # "Argument"
        # "Set Front Panel Open or Closed\n(Usage: \"UI: Front Panel State >> Open|Close\")"
        n61 = Unbundle By Name(w162) -> ("Core.Current VI Reference"=w161:refnum<vi>)
        n62 = case shown="\"Open\", \"Standard\", Default" w160 {
          tunnel: w164 -> [w172 w187 w198 w211 w224]
          tunnel: [w174 w188 w200 w213 w226] -> w163
          tunnel: w161 -> [w173 w185 w199 w212 w225]
          frame "Open", "Standard", Default {
            w167 = T2."Standard" ("State")
            n63 = property class="VI"(reference=w173, error in=w172) -> (reference out=w170:refnum<vi>, error out=w171:errorcluster, "FP.State"=w169:T2)
            n64 = Not Equal?(x=w169, y=w167) -> (x != y?=w168:bool)
            n65 = case shown="True" w168 {
              tunnel: [w178 w180] -> w174
              tunnel: w171 -> [w177 w180]
              tunnel: w170 -> [w176 _]
              tunnel: w167 -> [w175 _]
              frame True {
                n66 = invoke class="VI" method="FP.Open"(reference=w176, error in=w177, "Activate"=TRUE, "State"=w175) -> (error out=w178:errorcluster)  [unwired: 1 in, 4 out]
              }
              frame False {
              }
            }
          }
          frame "Close", "Closed" {
            n67 = property class="VI"(reference=w185, error in=w187) -> (reference out=w184:refnum<vi>, error out=w186:errorcluster, "FP.State"=w182:T2)
            n68 = Not Equal?(x=w182, y=T2."Closed" ("Front Panel Window:State")) -> (x != y?=w181:bool)
            n69 = case shown="True" w181 {
              tunnel: [w189 w192] -> w188
              tunnel: w186 -> [w189 w191]
              tunnel: w184 -> [_ w190]
              frame False {
              }
              frame True {
                n70 = invoke class="VI" method="FP.Close"(reference=w190, error in=w191) -> (error out=w192:errorcluster)  [unwired: 1 in, 2 out]
              }
            }
          }
          frame "Hidden", "Hide" {
            w193 = T2."Hidden" ("State")
            n71 = property class="VI"(reference=w199, error in=w198) -> (reference out=w196:refnum<vi>, error out=w197:errorcluster, "FP.State"=w195:T2)
            n72 = Not Equal?(x=w195, y=w193) -> (x != y?=w194:bool)
            n73 = case shown="True" w194 {
              tunnel: [w204 w205] -> w200
              tunnel: w197 -> [w203 w205]
              tunnel: w196 -> [w202 _]
              tunnel: w193 -> [w201 _]
              frame True {
                n74 = invoke class="VI" method="FP.Open"(reference=w202, error in=w203, "State"=w201) -> (error out=w204:errorcluster)  [unwired: 2 in, 4 out]
              }
              frame False {
              }
            }
          }
          frame "Minimize", "Minimized" {
            w206 = T2."Minimized" ("State")
            n75 = property class="VI"(reference=w212, error in=w211) -> (reference out=w209:refnum<vi>, error out=w210:errorcluster, "FP.State"=w208:T2)
            n76 = Not Equal?(x=w208, y=w206) -> (x != y?=w207:bool)
            n77 = case shown="True" w207 {
              tunnel: [w217 w218] -> w213
              tunnel: w210 -> [w216 w218]
              tunnel: w209 -> [w215 _]
              tunnel: w206 -> [w214 _]
              frame True {
                n78 = invoke class="VI" method="FP.Open"(reference=w215, error in=w216, "State"=w214) -> (error out=w217:errorcluster)  [unwired: 2 in, 4 out]
              }
              frame False {
              }
            }
          }
          frame "Maximize", "Maximized" {
            w219 = T2."Maximized" ("State")
            n79 = property class="VI"(reference=w225, error in=w224) -> (reference out=w222:refnum<vi>, error out=w223:errorcluster, "FP.State"=w221:T2)
            n80 = Not Equal?(x=w221, y=w219) -> (x != y?=w220:bool)
            n81 = case shown="True" w220 {
              tunnel: [w230 w231] -> w226
              tunnel: w223 -> [w229 w231]
              tunnel: w222 -> [w228 _]
              tunnel: w219 -> [w227 _]
              frame True {
                n82 = invoke class="VI" method="FP.Open"(reference=w228, error in=w229, "State"=w227) -> (error out=w230:errorcluster)  [unwired: 2 in, 4 out]
              }
              frame False {
              }
            }
          }
        }
        n83 = call <vilib>:"Add State(s) to Queue__JKI_lib_State_Machine.vi"("State(s) in (\"\")"=w166) -> ("States Out"=w165:string)  [unwired: 14 in]
      }
      frame "UI: Front Panel Size" {
        w232 = TRUE  # Subpanel Run?
        n84 = Unbundle By Name(w237) -> ("Core.Current VI Reference"=w236:refnum<vi>)
        n85 = case shown="True" w232 {
          tunnel: w236 -> [w243 _]
          tunnel: T4 {"Left"=4, "Top"=4, "Right"=1606, "Bottom"=996} ("Front Panel Window:Panel Bounds") -> [w242 _]
          tunnel: w234 -> [w241 w244]
          tunnel: [w240 w244] -> w233
          frame False {
            n86 = property class="VI"(reference=w243, error in=w241, "Front Panel.PanelBounds"=w242) -> (error out=w240:errorcluster)  [unwired: 1 out]
          }
          frame True {
          }
        }
        n87 = call <vilib>:"Add State(s) to Queue__JKI_lib_State_Machine.vi"("State(s) in (\"\")"=w239) -> ("States Out"=w238:string)  [unwired: 14 in]
      }
      frame "---------- Macro ----------" {
        # "Do not put any code in this frame.\n(It is a separator no-op. You can make a copy of this frame to create a new Macro frame)"
        n88 = call <vilib>:"Add State(s) to Queue__JKI_lib_State_Machine.vi"("State(s) in (\"\")"=w248) -> ("States Out"=w247:string)  [unwired: 14 in]
      }
      frame "Macro: Initialize" {
        w249 = "Data: Initialize\nInitialize Core Data\nUI: Initialize\nUI: Front Panel State >> Open"  # Data: Initialize Initialize Core Data UI: Initialize UI: Front Panel State >> Open
        # "Initialization Macro\n(This is called once, when the VI starts)"
        n89 = call <vilib>:"Add State(s) to Queue__JKI_lib_State_Machine.vi"("State(s) in Front (\"\")"=w249, "State(s) in (\"\")"=w253) -> ("States Out"=w252:string)  [unwired: 13 in]
      }
      frame "Macro: Exit" {
        # "Exit Macro\n(This is called once, when the VI exits)"
        n90 = Unbundle By Name(w268) -> ("Core.Close Panel on Exit?"=w267:bool)
        n91 = Unregister For Events(event registration refnum=w261, error in=w260) -> (error out=w259:errorcluster)
        n92 = call "Feedback Notifier.vi"("error in (no error)"=w259, "Action"=enum16{"Create", "Get", "Destroy"}."Get") -> ("error out"=w256:errorcluster, "notifier out"=w257:refnum<notifier>)  [unwired: 8 in]
        n93 = Send Notification(notification=TRUE, notifier=w257, error in (no error)=w256) -> (error out=w255:errorcluster)  [unwired: 1 out]
        n94 = Select(t="UI: Front Panel State >> Close", s=w267, f="") -> (s? t:f=w264:string)
        n95 = call <vilib>:"Add State(s) to Queue__JKI_lib_State_Machine.vi"("State(s) in (\"\")"=w264, "State(s) at Back (\"\")"="Data: Cleanup\nExit") -> ("States Out"=w262:string)  [unwired: 13 in]
        n96 = call <vilib>:"Add State(s) to Queue__JKI_lib_State_Machine.vi"("State(s) in Front (\"\")"=w262, "State(s) in (\"\")"=w270) -> ("States Out"=w269:string)  [unwired: 13 in]
      }
      frame "---------- New Category ----------" {
        # "Template Separator\n(You can make a copy of, or modify, this frame)"
        n97 = call <vilib>:"Add State(s) to Queue__JKI_lib_State_Machine.vi"("State(s) in (\"\")"=w274) -> ("States Out"=w273:string)  [unwired: 14 in]
      }
      frame "Save Configuration" {
        n98 = Unbundle By Name(w284) -> ("connection reference"=w278:T5, "Project ID"=w282:refnum<vi>, "Remark"=w281:refnum<vi>, "Controls[]"=w280:refnum<vi>[])  [unwired: 1 out]
        n99 = Build Array (concatenate)(w282, w281, w280) -> (w279:refnum<vi>[])
        n100 = call "Update Project Config.vi"("error in (no error)"=w283, "Array"=w279, "Refnum in"=w278) -> ("error out"=w276:errorcluster)  [unwired: 8 in]
        n101 = case shown="No Error" w276 {
          selector: w276 -> [w287 w288]
          tunnel: [w287 w289] -> w275
          frame No Error {
            n102 = call "Display Message to User3"() -> ()  [unwired: 10 in, 2 out]
          }
          frame Error {
            n103 = Unbundle By Name(w288) -> ("code"=w290:i32)
            n104 = case shown="-2147217900" w290 {
              tunnel: [w291 w292] -> w289
              tunnel: w288 -> [w291 w293]
              frame 0, Default {
              }
              frame -2147217900 {
                n105 = call <vilib>:"Clear Errors.vi"("error in (no error)"=w293) -> ("error out"=w292:errorcluster)  [unwired: 5 in, 1 out]
                n106 = call "Display Message to User2"() -> ()  [unwired: 10 in, 2 out]
              }
            }
          }
        }
        n107 = call <vilib>:"Add State(s) to Queue__JKI_lib_State_Machine.vi"("State(s) in (\"\")"=w286, "State(s) at Back (\"\")"="UI: Update ProjID" ("State(s) at Back (\"\")")) -> ("States Out"=w285:string)  [unwired: 13 in]
      }
      frame "Get Configuration" {
        # "Your code here.\n(You can make a copy of, or modify, this frame)"
        n108 = Unbundle By Name(w314) -> ("Project ID"=w303:refnum<vi>, "connection reference"=w313:T5)
        n109 = property class="CmbBox"(reference=w303) -> ("Value"=w312:string)  [unwired: 1 in, 2 out]
        n110 = Format Into String(format string="where ProjectID='%s'", w312) -> (resulting string=w310:string)  [unwired: 2 in, 1 out]
        n111 = call <vilib>:"DB Tools Select Data.vi"("condition"=w310, "error in (no error)"=w308, "table"="ProjectConfig", "connection reference"=w313) -> ("error out"=w305:errorcluster, "data"=w307:variant[][])  [unwired: 2 in, 1 out]
        n112 = Variant To Data(error in=w305, type=string[][] [], Variant=w307) -> (data=w302:string[][], error out=w304:errorcluster)
        n113 = Index Array(array=w302, index (row)=0) -> (element=w300:string[])  [unwired: 1 in]
        n114 = Delete From Array(array=w300, length=2, index=32) -> (deleted portion=w295:string[], array with subset deleted=w297:string[])
        n115 = Index Array(array=w295) -> (element #2=w294:string)  [unwired: 2 in, 1 out]
        n116 = Array To Cluster(array=w297) -> (cluster=w296:T8)
        n117 = call <vilib>:"Add State(s) to Queue__JKI_lib_State_Machine.vi"("State(s) in (\"\")"=w316) -> ("States Out"=w315:string)  [unwired: 14 in]
        n118 = local write "Remark"(w294) -> ()
        n119 = local write "Configuration"(w296) -> ()
      }
      frame "Delete ProjectID" {
        n120 = call "Display Message to User5"("error in (no error)"=w318) -> ("error out"=w317:errorcluster, "OK"=w319:bool)  [unwired: 9 in]
        n121 = case shown="True" w319 {
          tunnel: w324 -> [_ w335]
          tunnel: w317 -> [w325 w329]
          tunnel: [w325 w326] -> w320
          frame False {
          }
          frame True {
            n122 = Unbundle By Name(w335) -> ("connection reference"=w334:T5)
            n123 = Format Into String(format string="where ProjectID ='%s'", error in=w329, "Project ID") -> (resulting string=w330:string, error out=w328:errorcluster)  [unwired: 1 in]
            n124 = call <vilib>:"DB Tools Delete Data.vi"("condition"=w330, "error in (no error)"=w328, "table"="ProjectConfig", "connection reference"=w334) -> ("error out"=w327:errorcluster)  [unwired: 6 in, 1 out]
            n125 = case shown="No Error" w327 {
              selector: w327 -> [w336 w338]
              tunnel: [w336 w338] -> w326
              frame No Error {
                n126 = call "Display Message to User"() -> ()  [unwired: 10 in, 2 out]
                n127 = local write "Project ID"("") -> ()
              }
              frame Error {
                n128 = call "Display Message to User4"() -> ()  [unwired: 10 in, 2 out]
              }
            }
          }
        }
        n129 = call <vilib>:"Add State(s) to Queue__JKI_lib_State_Machine.vi"("State(s) in (\"\")"=w322, "State(s) at Back (\"\")"="UI: Update ProjID" ("State(s) at Back (\"\")")) -> ("States Out"=w323:string)  [unwired: 13 in]
      }
    }
  }
